vi "LABV_Maes_Daan_DiscretePID.vi"() -> ()   [LabVIEW 2021]
panel:
  out "Stuurwaarde systeem na PID":dbl[](graph)
  in  "Tab Control":T1(tab)
  in  "Nr .......x":dbl=3.0
  in  "Nr ......x.":dbl=1.0
  in  "Nr ....x..":dbl=8.0
  in  "Kr":dbl=0.05
  in  "tau I":dbl=40.0
  in  "tau D":dbl=1.0
  in  "T":dbl=15.0
  in  "Startwaarde uitgang":dbl format="%#_13g"
  in  "Setwaarde":dbl=10.0
  in  "Hoeveel keer is systeem sneller":i32=10
  in  "Aantal uit te voeren cycli":i32=25
  out "Open lus versterking":dbl
  out "c":dbl
  out "b":dbl
  out "a":dbl
  out "Combinatie van beide signalen":cluster{i32[], dbl[]}[](graph)
  out "Uitgang systeem":dbl[](graph)
  # "Discrete PID regelaar"
  # "Daan Maes"
  # "Studentennummer"
  # "1952813"
  # "Regelaarsinstelling"
  # "Instelling systeem"
  # "Berekende waardes"
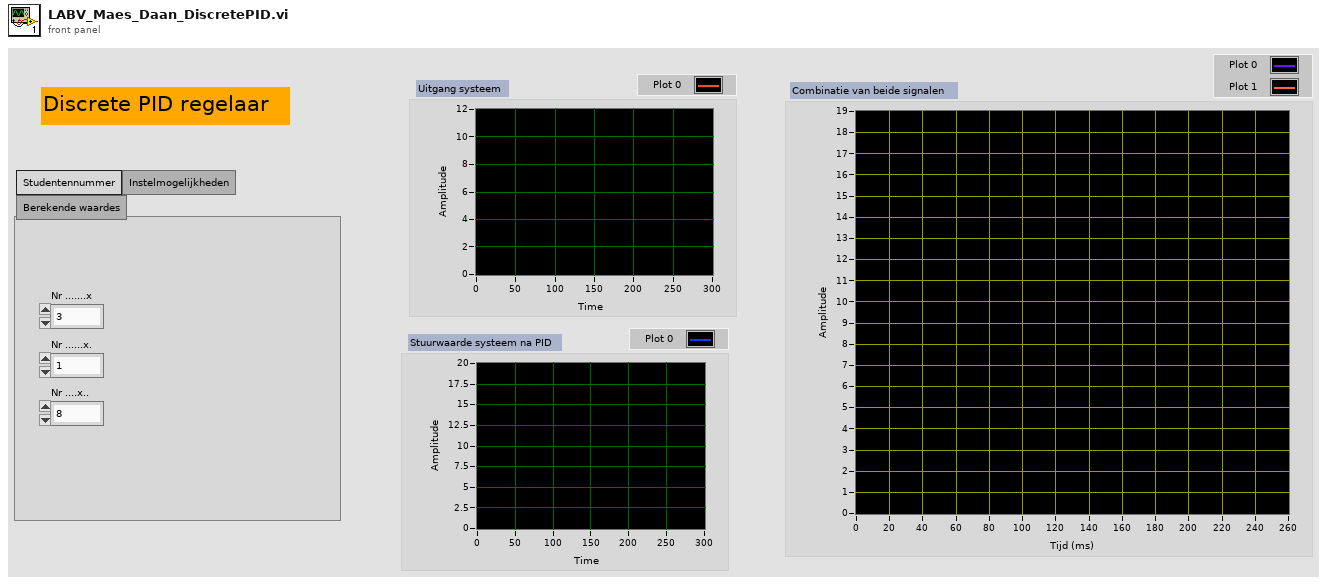
[diagram p1: front panel]
types:
  T1 = enum32{"Studentennummer", "Instelmogelijkheden", "Berekende waardes"}
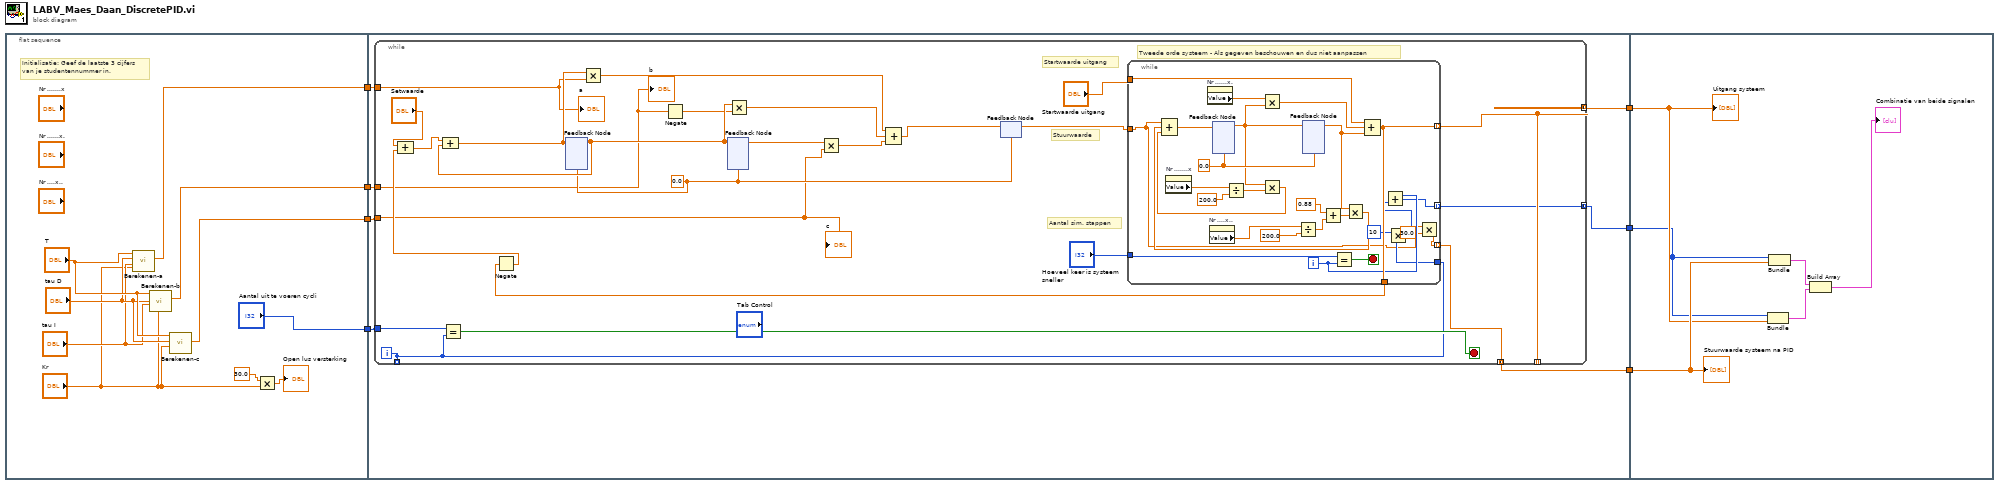
[diagram p0: block diagram]
diagram:
  n1 = flat-sequence {
    tunnel: ["Aantal uit te voeren cycli"] -> w7
    tunnel: [w13] -> w3
    tunnel: [w12] -> w2
    tunnel: [w11] -> w1
    tunnel: w7 -> [w24]
    tunnel: [w23] -> w6
    tunnel: [w22] -> w5
    tunnel: [w21] -> w4
    tunnel: w3 -> [w20]
    tunnel: w2 -> [w19]
    tunnel: w1 -> [w18]
    tunnel: w6 -> [w82]
    tunnel: w5 -> [w83]
    tunnel: w4 -> [w78]
    frame #0 {
      # "Initialisatie: Geef de laatste 3 cijfers\nvan je studentennummer in."
      n2 = call "Berekenen-a.vi"("K"="Kr", "Ti"="tau I", "Td"="tau D", "T"="T") -> ("A"=w13:dbl)  [unwired: 7 in]
      n3 = call "Berekenen-b.vi"("K"="Kr", "Ti"="tau I", "Td"="tau D", "T"="T") -> ("B"=w12:dbl)  [unwired: 7 in]
      n4 = call "Berekenen-c.vi"("K"="Kr", "Td"="tau D", "T"="T") -> ("C"=w11:dbl)  [unwired: 8 in]
      n5 = Multiply(x=30.0, y="Kr") -> (x*y=→"Open lus versterking":dbl)
    }
    frame #1 {
      n6 = while {
        tunnel: w24 -> [w38]
        tunnel: [w32] -> w23 mode=concatenating
        tunnel: [w30] -> _ mode=indexing
        tunnel: [w32] -> _ mode=indexing
        tunnel: [w31] -> w22 mode=concatenating
        tunnel: [w29] -> w21 mode=concatenating
        tunnel: w20 -> [w27]
        tunnel: w19 -> [w26]
        tunnel: w18 -> [w25]
        i -> [w30]
        stop <- w37 stop-if-true
        w28 = 0.0 ("Nr ....x..")
        # "Aantal sim. stappen"
        # "Startwaarde uitgang"
        # "Tweede orde systeem - Als gegeven beschouwen en dus niet aanpassen"
        # "Stuurwaarde"
        n7 = Equal?(x=w38, y=w30) -> (x = y?=w37:bool)
        n8 = feedback #1(w28) -> (w47:dbl)
        n9 = Negate(x=w26) -> (-x=w36:dbl)
        n10 = feedback #2(w28) -> (w43:dbl)
        n11 = feedback-in #2(w47) -> ()
        n12 = Multiply(x=w47, y=w36) -> (x*y=w45:dbl)
        n13 = Multiply(x=w43, y=w25) -> (x*y=w42:dbl)
        n14 = feedback #3(w28) -> (w33:dbl)
        n15 = while {
          tunnel: w33 -> [w51]
          tunnel: [w58] -> w32 mode=indexing
          tunnel: "Startwaarde uitgang" -> [w60]
          tunnel: "Hoeveel keer is systeem sneller" -> [w59]
          tunnel: [w58] -> w35
          tunnel: [w52] -> w31 mode=indexing
          tunnel: w30 -> [w55]
          tunnel: [w53] -> w29 mode=indexing
          i -> [w57]
          stop <- w77 stop-if-true
          w76 = 0.0 ("Nr ....x..")
          n16 = property on="Nr .......x" class="DigNum (strict)"() -> ("Value"=w68:dbl)  [unwired: 2 in, 2 out]
          n17 = property on="Nr ......x." class="DigNum (strict)"() -> ("Value"=w72:dbl)  [unwired: 2 in, 2 out]
          n18 = property on="Nr ....x.." class="DigNum (strict)"() -> ("Value"=w66:dbl)  [unwired: 2 in, 2 out]
          n19 = feedback #4(w76) -> (w71:dbl)
          n20 = Divide(x=w68, y=200.0) -> (x/y=w67:dbl)
          n21 = Multiply(x=w72, y=w71) -> (x*y=w70:dbl)
          n22 = Multiply(x=w71, y=w67) -> (x*y=w75:dbl)
          n23 = Divide(x=w66, y=200.0) -> (x/y=w64:dbl)
          n24 = feedback #5(w76) -> (w61:dbl)
          n25 = feedback-in #5(w71) -> ()
          n26 = Add(x=0.88 ("Nr ....x.."), y=w64) -> (x+y=w62:dbl)
          n27 = Equal?(x=w59, y=w57) -> (x = y?=w77:bool)
          n28 = Multiply(x=w61, y=w62) -> (x*y=w73:dbl)
          n29 = Compound Arithmetic op=ADD(w51, w73, w75) -> (w74:dbl)
          n30 = feedback-in #4(w74) -> ()
          n31 = Compound Arithmetic op=ADD(w60, w70, w61) -> (w58:dbl)
          n32 = Multiply(x=10, y=w55) -> (x*y=w56:i32)
          n33 = Add(x=w57, y=w56) -> (x+y=w53:i32)
          n34 = Multiply(x=w51, y=30.0) -> (x*y=w52:dbl)
        }
        n35 = Negate(x=w35) -> (-x=w40:dbl)
        n36 = Compound Arithmetic op=ADD("Setwaarde", w40) -> (w41:dbl)
        n37 = Compound Arithmetic op=ADD(w41, w47) -> (w44:dbl)
        n38 = feedback-in #1(w44) -> ()
        n39 = Multiply(x=w44, y=w27) -> (x*y=w46:dbl)
        n40 = Compound Arithmetic op=ADD(w46, w45, w42) -> (w34:dbl)
        n41 = feedback-in #3(w34) -> ()
        "a" <- w27
        "b" <- w26
        "c" <- w25
      }
    }
    frame #2 {
      n42 = Bundle(w78, w82) -> (w80:cluster{i32[], dbl[]})  [unwired: 1 in]
      n43 = Bundle(w78, w83) -> (w81:cluster{i32[], dbl[]})  [unwired: 1 in]
      n44 = Build Array(w81, w80) -> (→"Combinatie van beide signalen":cluster{i32[], dbl[]}[])
      "Uitgang systeem" <- w82
      "Stuurwaarde systeem na PID" <- w83
    }
  }
